vi "RTS Relay 2 Startup.vi"(11 "Station 1-8 Data in":T1 {"Station Slide"."Chamber 1-1"."Start Time" format="%<%X\n%x>T"; "Station Slide"."Chamber 1-1"."End Time" format="%<%X\n%x>T"; "Station Slide"."Time Count (s)" format="%.2f"; "Station Cab"."Chamber 1-1"."Start Time" format="%<%X\n%x>T"; "Station Cab"."Chamber 1-1"."End Time" format="%<%X\n%x>T"; "Station Cab"."Time Count (s)" format="%.2f"; "Station Freezer"."Chamber 1-1"."Start Time" format="%<%X\n%x>T"; "Station Freezer"."Chamber 1-1"."End Time" format="%<%X\n%x>T"; "Station Freezer"."Time Count (s)" format="%.2f"}) -> (3 "Run Door Ops":bool)   [LabVIEW 2016]
uses:
  Type Definitions/RTS Station Relay Ops.ctl
  Type Definitions/RTS Door Opener Indicator.ctl
  Type Definitions/RTS Door Ops Client.ctl
  Type Definitions/RTS Door Opening Schedule.ctl
  Type Definitions/RTS Door Ops Sequence.ctl
panel:
  # "Chamber Conditions:"
  # "Chamber Conditions:"
  # "Chamber Conditions:"
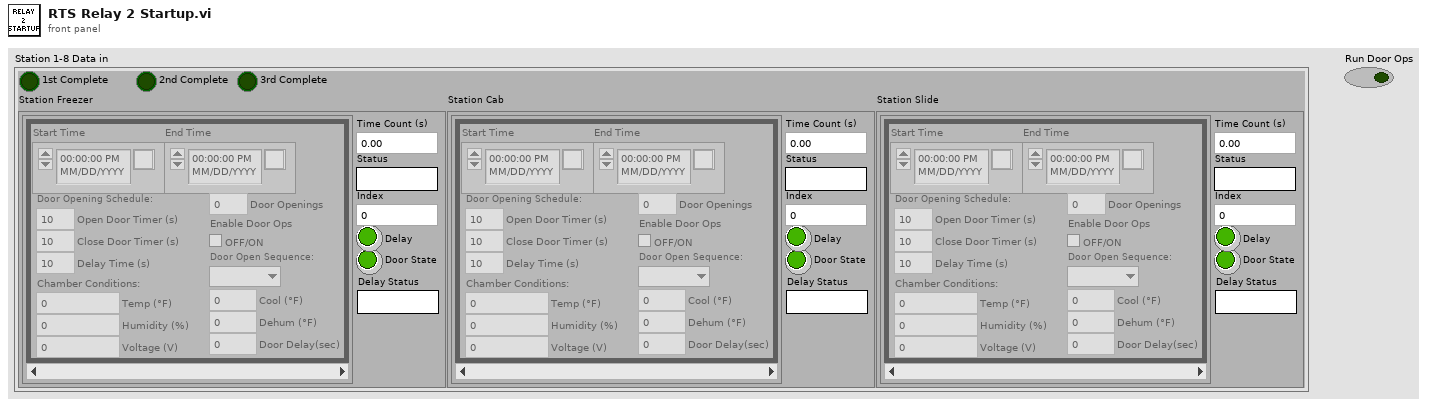
[diagram p1: front panel]
types:
  T1 = typedef "RTS Station Relay Ops.ctl" = cluster{"Station Freezer":T2, "Station Cab":T2, "Station Slide":T2, "1st Complete":bool, "2nd Complete":bool, "3rd Complete":bool}
  T2 = typedef "RTS Door Opener Indicator.ctl" = cluster{"Time Count (s)":dbl, "Status":string, "Door State":bool, "Delay":bool, "Chamber 1-1":T3[], "Index":i32, "Delay Status":string}
  T3 = typedef "RTS Door Ops Client.ctl" = cluster{"End Time":timestamp, "Start Time":timestamp, "Door Opening Schedule:":T4, "Enable Door Ops":bool, "Door Openings":u32, "Temp (°F)":dbl, "Humidity (%)":dbl, "Voltage (V)":dbl, "Door Open Sequence:":T5, "Door Delay(sec)":dbl, "Dehum (°F)":dbl, "Cool (°F)":dbl}
  T4 = typedef "RTS Door Opening Schedule.ctl" = cluster{"Open Door Timer (s)":dbl, "Delay Time (s)":dbl, "Close Door Timer (s)":dbl}
  T5 = typedef "RTS Door Ops Sequence.ctl" = enum16{"", "1st", "2nd", "3rd"}
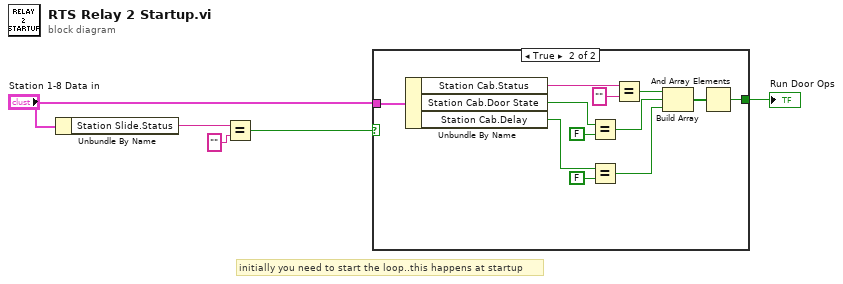
[diagram p0: block diagram]
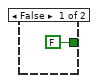
[diagram p2: hidden frame]
diagram:
  # "initially you need to start the loop..this happens at startup"
  n1 = Unbundle By Name("Station 1-8 Data in") -> ("Station Slide.Status"=w3:string)
  n2 = Equal?(x=w3, y="") -> (x = y?=w5:bool)
  n3 = case shown="True" w5 {
    tunnel: [FALSE w8] -> w1
    tunnel: "Station 1-8 Data in" -> [_ w7]
    frame False {
    }
    frame True {
      n4 = Unbundle By Name(w7) -> ("Station Cab.Status"=w11:string, "Station Cab.Door State"=w10:bool, "Station Cab.Delay"=w9:bool)
      n5 = Equal?(x=w10, y=FALSE) -> (x = y?=w14:bool)
      n6 = Equal?(x=w9, y=FALSE) -> (x = y?=w13:bool)
      n7 = Equal?(x=w11, y="") -> (x = y?=w15:bool)
      n8 = Build Array(w15, w14, w13) -> (w12:bool[])
      n9 = And Array Elements(Boolean array=w12) -> (logical AND=w8:bool)
    }
  }
  "Run Door Ops" <- w1
